vi "Handle Result.vi"(8 "error in (no error)":errorcluster, 10 "Result":T1={"Name"="", "Message"="", "Description"="", "Status"=enum."Passed", "Result Type"=enum."Test Suite", "Execution Time"=0.0}, 11 "Text Report In":refnum<class "Text Report.lvclass">) -> (0 "error out":errorcluster, 3 "Text Report Out":refnum<class "Text Report.lvclass">)   [LabVIEW 2020, in "Reports.lvlib" / "Text Report.lvclass"]
uses:
  Text Report.lvclass
  Core/Result/Result.ctl
  Core/Result/Status.ctl
  Core/Result/Type.ctl
  Text Report.lvclass/Text Report.ctl
  Core/Result/Result.lvlib
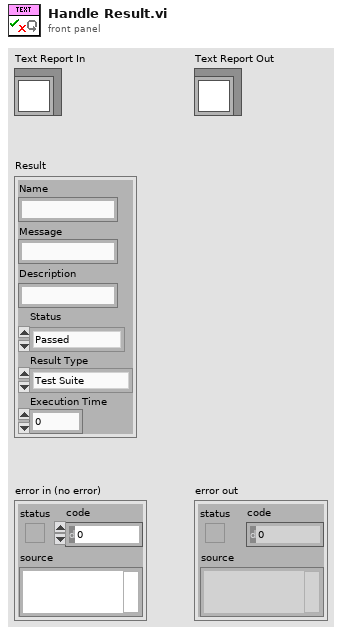
[diagram p1: front panel]
types:
  T1 = typedef "Result.lvlib/Result.ctl" = cluster{"Name":string, "Message":string, "Description":string, "Status":T2, "Result Type":T3, "Execution Time":dbl}
  T2 = typedef "Result.lvlib/Status.ctl" = enum16{"", "Passed", "Failed", "Error", "Skipped", "Setup Error", "Broken", "Teardown Error"}
  T3 = typedef "Result.lvlib/Type.ctl" = enum16{"Test Case", "Test Suite", "Test Run", "Pass", "Fail", "Skip", "Pass if", "Fail if", "Pass if Error", "Fail if Error", "Pass if Equal", "Fail if Equal"}
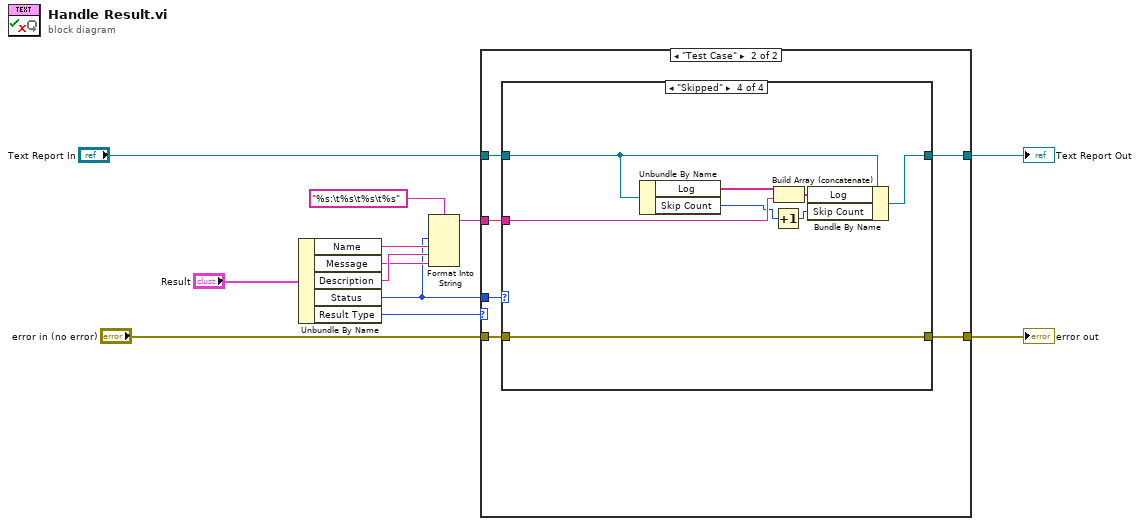
[diagram p0: block diagram]
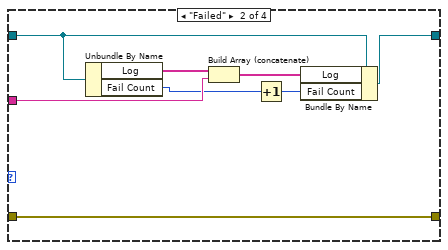
[diagram p4: hidden frame]
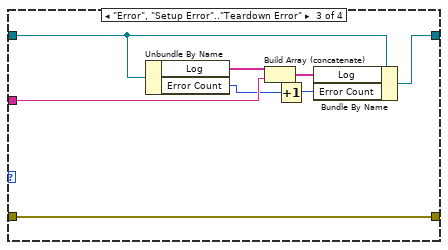
[diagram p5: hidden frame]
diagram:
  n1 = Unbundle By Name("Result") -> ("Name"=w8:string, "Message"=w6:string, "Description"=w7:string, "Status"=w4:T2, "Result Type"=w1:T3)
  n2 = Format Into String(format string="%s:\t%s\t%s\t%s", w4, w8, w7, w6) -> (resulting string=w5:string)  [unwired: 2 in, 1 out]
  n3 = case shown="\"Test Case\"" w1 {
    tunnel: "error in (no error)" -> [w13 w20]
    tunnel: [w13 w19] -> w11
    tunnel: w5 -> [_ w18]
    tunnel: w4 -> [_ w17]
    tunnel: "Text Report In" -> [w14 w16]
    tunnel: [w14 w15] -> w2
    frame Default {
    }
    frame "Test Case" {
      n4 = case shown="\"Skipped\"" w17 {
        tunnel: w20 -> [w22 w30 w38 w46]
        tunnel: [w22 w30 w38 w46] -> w19
        tunnel: w18 -> [_ w29 w37 w45]
        tunnel: w16 -> [w21 w27 w35 w43]
        tunnel: [w21 w25 w33 w41] -> w15
        frame "", Default {
        }
        frame "Failed" {
          n5 = Unbundle By Name(w27) -> ("Log"=w28:string[], "Fail Count"=w23:i32)
          n6 = Build Array (concatenate)(w28, w29) -> (w26:string[])
          n7 = Increment(x=w23) -> (x+1=w24:i32)
          n8 = Bundle By Name(cluster=w27, "Log"=w26, "Fail Count"=w24) -> (w25:refnum<class "Text Report.lvclass">)
        }
        frame "Error", "Setup Error".."Teardown Error" {
          n9 = Unbundle By Name(w35) -> ("Log"=w36:string[], "Error Count"=w31:i32)
          n10 = Build Array (concatenate)(w36, w37) -> (w34:string[])
          n11 = Increment(x=w31) -> (x+1=w32:i32)
          n12 = Bundle By Name(cluster=w35, "Log"=w34, "Error Count"=w32) -> (w33:refnum<class "Text Report.lvclass">)
        }
        frame "Skipped" {
          n13 = Unbundle By Name(w43) -> ("Log"=w44:string[], "Skip Count"=w39:i32)
          n14 = Increment(x=w39) -> (x+1=w40:i32)
          n15 = Build Array (concatenate)(w44, w45) -> (w42:string[])
          n16 = Bundle By Name(cluster=w43, "Log"=w42, "Skip Count"=w40) -> (w41:refnum<class "Text Report.lvclass">)
        }
      }
    }
  }
  "error out" <- w11
  "Text Report Out" <- w2
